vi "New Pickup.vi"(8 "New Lift Height":dbl, 9 "Distance Up":dbl=28.0, 10 "Distance Down":dbl=28.0, 11 "Original State":string) -> (3 "New State":string)   [LabVIEW 2014]
uses:
  Begin/Global Variables.vi
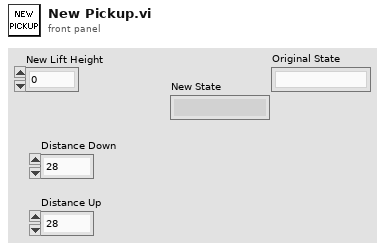
[diagram p1: front panel]
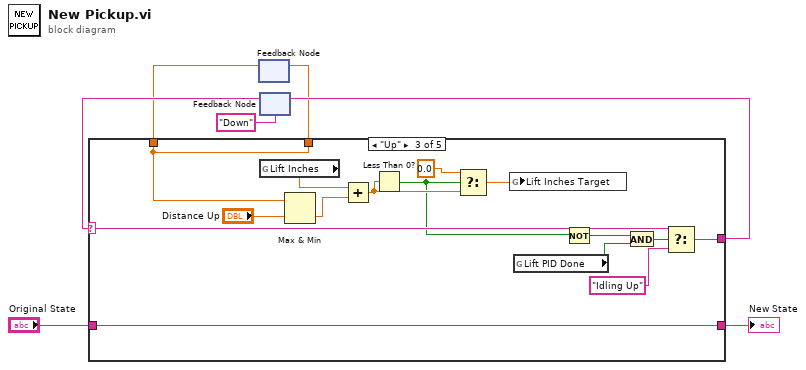
[diagram p0: block diagram]
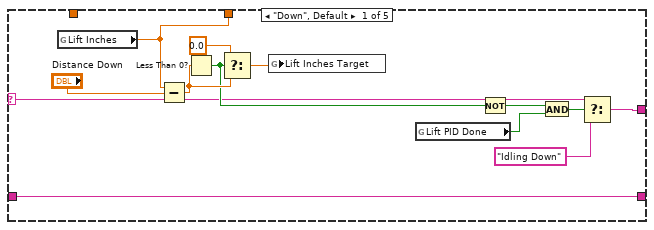
[diagram p2: hidden frame]
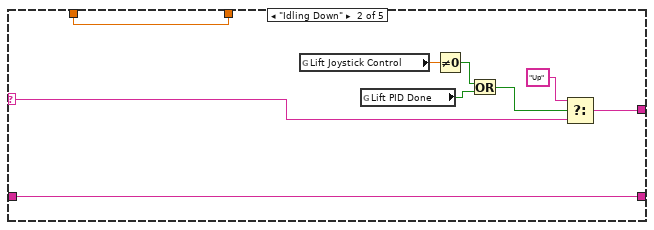
[diagram p3: hidden frame]
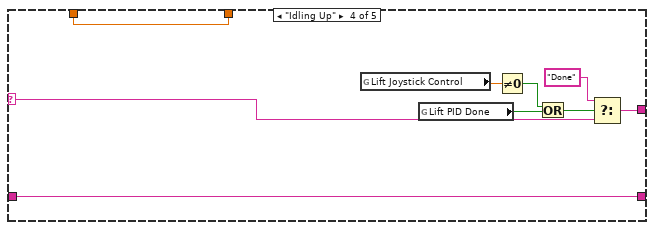
[diagram p4: hidden frame]
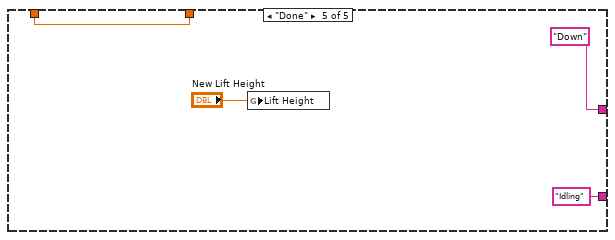
[diagram p5: hidden frame]
diagram:
  n1 = feedback #1() -> (w1:dbl)  [unwired: 1 in]
  n2 = feedback #2("Down") -> (w7:string)
  n3 = case shown="\"Up\"" w7 {
    selector: w7 -> [w10 w25 w38 w47 _]
    tunnel: [w12 w24 w37 w48 "Down" ("t")] -> w6
    tunnel: [w9 w22 w31 w46 "Idling" ("t")] -> w4
    tunnel: "Original State" -> [w9 w22 w31 w46 _]
    tunnel: [w8 w21 w30 w45 w54] -> w2
    tunnel: w1 -> [_ w21 w30 w45 w54]
    frame "Down", Default {
      n4 = global read "Global Variables.vi" "Lift Inches"() -> (w8:dbl)
      n5 = Subtract(x=w8, y="Distance Down") -> (x-y=w19:dbl)
      n6 = Less Than 0?(x=w19) -> (x < 0?=w14:bool)
      n7 = Select(t=0.0, s=w14, f=w19) -> (s? t:f=w17:dbl)
      n8 = global write "Global Variables.vi" "Lift Inches Target"(w17) -> ()
      n9 = global read "Global Variables.vi" "Lift PID Done"() -> (w16:bool)
      n10 = Not(x=w14) -> (.not. x?=w15:bool)
      n11 = And(x=w15, y=w16) -> (x .and. y?=w13:bool)
      n12 = Select(t=w10, s=w13, f="Idling Down") -> (s? t:f=w12:string)
    }
    frame "Idling Down" {
      n13 = global read "Global Variables.vi" "Lift Joystick Control"() -> (w28:dbl)
      n14 = global read "Global Variables.vi" "Lift PID Done"() -> (w29:bool)
      n15 = Not Equal To 0?(x=w28) -> (x != 0?=w27:bool)
      n16 = Or(x=w27, y=w29) -> (x .or. y?=w26:bool)
      n17 = Select(t="Up", s=w26, f=w25) -> (s? t:f=w24:string)
    }
    frame "Up" {
      n18 = global read "Global Variables.vi" "Lift Inches"() -> (w43:dbl)
      n19 = Max & Min(x=w30, y="Distance Up") -> (min(x,y)=w39:dbl)  [unwired: 1 out]
      n20 = Add(x=w43, y=w39) -> (x+y=w44:dbl)
      n21 = Less Than 0?(x=w44) -> (x < 0?=w34:bool)
      n22 = Select(t=0.0, s=w34, f=w44) -> (s? t:f=w42:dbl)
      n23 = global write "Global Variables.vi" "Lift Inches Target"(w42) -> ()
      n24 = global read "Global Variables.vi" "Lift PID Done"() -> (w36:bool)
      n25 = Not(x=w34) -> (.not. x?=w35:bool)
      n26 = And(x=w35, y=w36) -> (x .and. y?=w33:bool)
      n27 = Select(t=w38, s=w33, f="Idling Up") -> (s? t:f=w37:string)
    }
    frame "Idling Up" {
      n28 = global read "Global Variables.vi" "Lift Joystick Control"() -> (w52:dbl)
      n29 = global read "Global Variables.vi" "Lift PID Done"() -> (w53:bool)
      n30 = Not Equal To 0?(x=w52) -> (x != 0?=w51:bool)
      n31 = Or(x=w51, y=w53) -> (x .or. y?=w50:bool)
      n32 = Select(t="Done", s=w50, f=w47) -> (s? t:f=w48:string)
    }
    frame "Done" {
      n33 = global write "Global Variables.vi" "Lift Height"("New Lift Height") -> ()
    }
  }
  "New State" <- w4
  n34 = feedback-in #1(w2) -> ()
  n35 = feedback-in #2(w6) -> ()
